vi "Change Flame Level - Next.vi"(7 "Limit?":bool, 8 "error in":errorcluster, 9 "Increment?":bool, 10 "Handshake":refnum<notifier>, 11 "Boiler Queue in":refnum<queue>) -> (0 "error out":errorcluster)   [LabVIEW 2022 SP3, in "Boiler.lvlib"]
doc: "Choose the next command for the boiler after incrementing/decrementing the flame level of the boiler."
uses:
  Boiler.lvlib
  support/Message Queue/Message Cluster.ctl
  support/Message Queue/Message Queue.lvlib
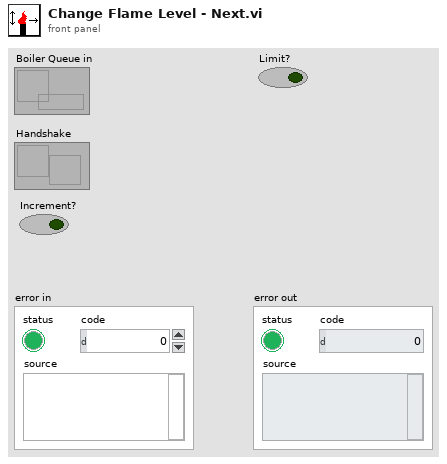
[diagram p1: front panel]
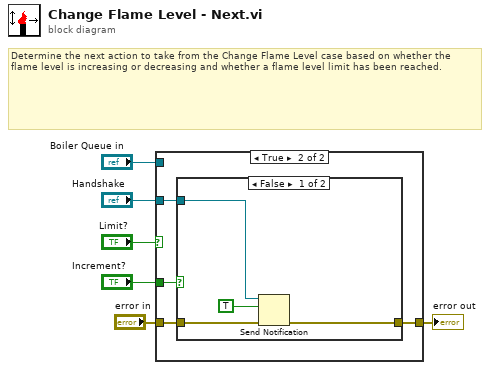
[diagram p0: block diagram]
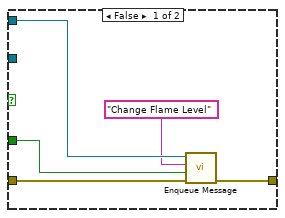
[diagram p2: hidden frame]
diagram:
  # "Determine the next action to take from the Change Flame Level case based on whether the flame level is increasing or decreasing and whether a flame level limit has been reached."
  n1 = case shown="True" "Limit?" {
    tunnel: "error in" -> [w11 w15]
    tunnel: [w10 w14] -> w2
    tunnel: "Increment?" -> [w9 w13]
    tunnel: "Boiler Queue in" -> [w8 _]
    tunnel: "Handshake" -> [_ w12]
    frame False {
      n2 = call "Enqueue Message.vi"("error in"=w11, "Message Data"=w9, "Message"="Change Flame Level", "Message Queue"=w8) -> ("error out"=w10:errorcluster)  [unwired: 6 in, 1 out]
    }
    frame True {
      n3 = case shown="False" w13 {
        tunnel: w15 -> [w19 w20]
        tunnel: [w18 w20] -> w14
        tunnel: w12 -> [w16 _]
        frame False {
          n4 = Send Notification(notification=TRUE ("Run Interlock"), notifier=w16, error in (no error)=w19) -> (error out=w18:errorcluster)  [unwired: 1 out]
        }
        frame True {
        }
      }
    }
  }
  "error out" <- w2
